vi "Instrument.Aerotech.Read Configuration.vi"(8 "error in (no error)":errorcluster, 11 "Instrument.Aerotech":refnum<class "Instrument.Aerotech.lvclass">) -> (0 "error out":errorcluster, 2 "Configuration":T1, 3 "Instrument.Aerotech out":refnum<class "Instrument.Aerotech.lvclass">)   [LabVIEW 2016, in "Instrument.Aerotech.lvclass"]
uses:
  Instrument.Aerotech.lvclass
  Typedefs/Instrument.Aerotech.Configuration--Cluster.ctl
  Instrument.Aerotech.lvclass/Instrument.Aerotech.ctl
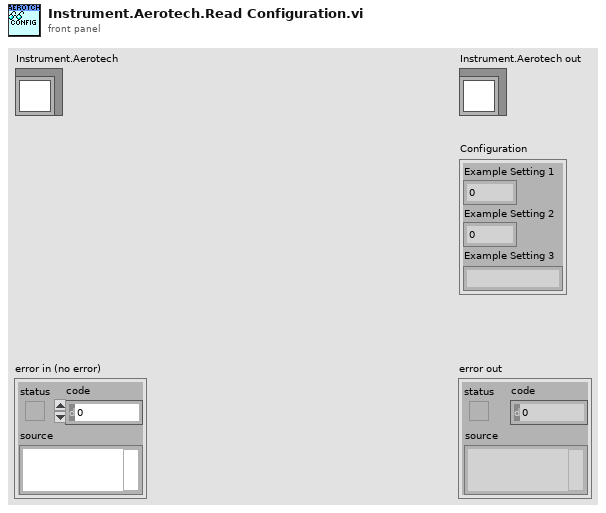
[diagram p1: front panel]
types:
  T1 = typedef "Instrument.Aerotech.lvclass/Instrument.Aerotech.Configuration--Cluster.ctl" = cluster{"Example Setting 1":dbl, "Example Setting 2":dbl, "Example Setting 3":string}
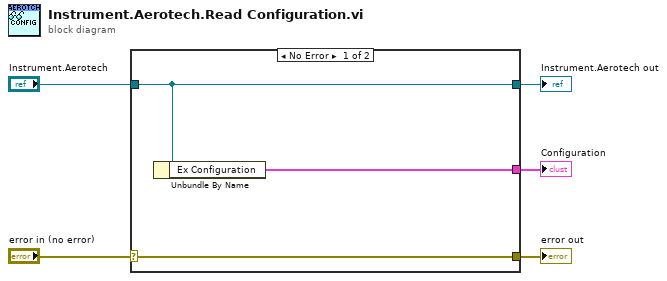
[diagram p0: block diagram]
diagram:
  n1 = case shown="No Error" "error in (no error)" {
    selector: "error in (no error)" -> [w8 w9]
    tunnel: [w8 w9] -> w4
    tunnel: [w7 w10] -> w2
    tunnel: "Instrument.Aerotech" -> [w7 w10]
    tunnel: [w6 _] -> w1
    frame No Error {
      n2 = Unbundle By Name(w7) -> ("Ex Configuration"=w6:T1)
    }
    frame Error {
    }
  }
  "error out" <- w4
  "Instrument.Aerotech out" <- w2
  "Configuration" <- w1
